vi "Write denude_.vi"(8 "error in (no error)":errorcluster, 10 "denude?":bool, 11 "Change Denuder State MSG in":refnum<class "Change Denuder State MSG.lvclass">) -> (0 "error out":errorcluster, 3 "Change Denuder State MSG out":refnum<class "Change Denuder State MSG.lvclass">)   [LabVIEW 2014, in "Controller.lvlib" / "Change Denuder State MSG.lvclass"]
uses:
  Change Denuder State MSG.lvclass
  Change Denuder State MSG.lvclass/Change Denuder State MSG.ctl
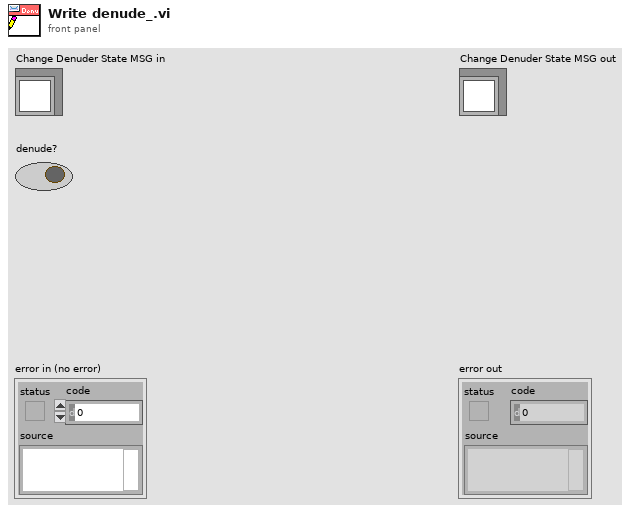
[diagram p1: front panel]
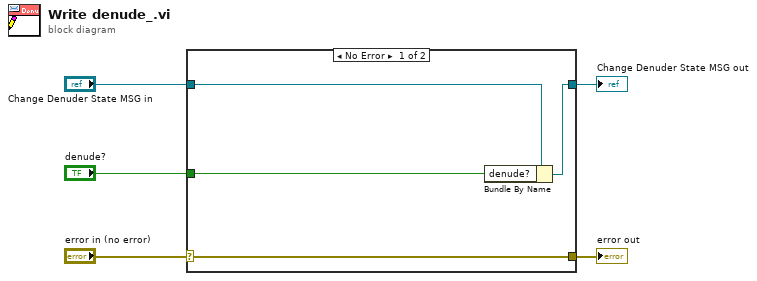
[diagram p0: block diagram]
diagram:
  n1 = case shown="No Error" "error in (no error)" {
    selector: "error in (no error)" -> [w9 w10]
    tunnel: [w9 w10] -> w4
    tunnel: [w7 w11] -> w2
    tunnel: "Change Denuder State MSG in" -> [w8 w11]
    tunnel: "denude?" -> [w6 _]
    frame No Error {
      n2 = Bundle By Name(cluster=w8, "denude?"=w6) -> (w7:refnum<class "Change Denuder State MSG.lvclass">)
    }
    frame Error {
    }
  }
  "error out" <- w4
  "Change Denuder State MSG out" <- w2
